vi "Support_Top_Level.vi"(8 "error in (no error)":errorcluster, 11 "AB_Dest_LLB in":refnum<class "AB_Dest_LLB.lvclass">) -> (0 "error out":errorcluster, 1 "displayTopLevel":bool, 2 "supportTopLevel":bool, 3 "AB_Dest_LLB out":refnum<class "AB_Dest_LLB.lvclass">)   [LabVIEW 2020, in "AB_Dest_LLB.lvclass"]
uses:
  <vilib>/AppBuilder/AB_Classes/Destination/Dest_LLB/AB_Dest_LLB.lvclass
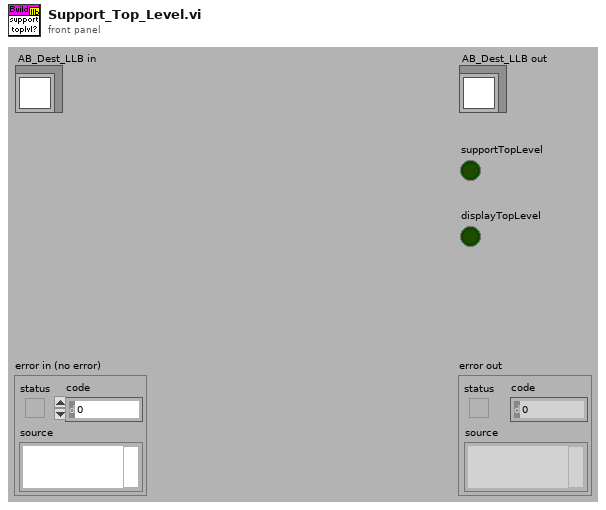
[diagram p1: front panel]
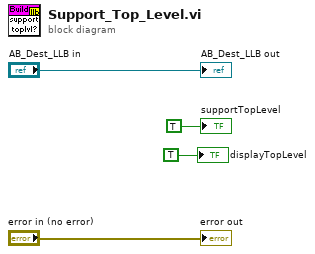
[diagram p0: block diagram]
diagram:
  "error out" <- "error in (no error)"
  "supportTopLevel" <- TRUE ("supportTopLevel")
  "AB_Dest_LLB out" <- "AB_Dest_LLB in"
  "displayTopLevel" <- TRUE ("supportTopLevel")
